vi "Stop AMC Queue.vi"(8 "error in (no error)":errorcluster, 11 "Model_AMC in":refnum<class "Model_AMC.lvclass">) -> (0 "error out":errorcluster, 2 "Exist CMD":string, 3 "Model_AMC out":refnum<class "Model_AMC.lvclass">)   [LabVIEW 2021, in "Model_AMC.lvclass"]
uses:
  Model_AMC.lvclass
  Model_AMC.lvclass/Model_AMC.ctl
  58014273-f04a-4b47-9aff-988d5dec622c.vi
  8ad511de-be0c-4148-9c49-af70c3a993ee.vi
  <vilib>/ActorFramework/Stop Msg/Stop Msg.lvclass
  <vilib>/ActorFramework/Actor/Actor.lvclass
  C:/Program Files (x86)/National Instruments/LabVIEW 2021/user.lib/John_Lib/AbstractActorTemplate/AbstractActorTemplate/UIActorTop.lvclass
  C:/Program Files (x86)/National Instruments/LabVIEW 2021/vi.lib/ActorFramework/Actor/Actor.lvclass
  C:/Program Files (x86)/National Instruments/LabVIEW 2021/project/Create Actor from Template/_Model_AMC/Model_AMC.lvclass
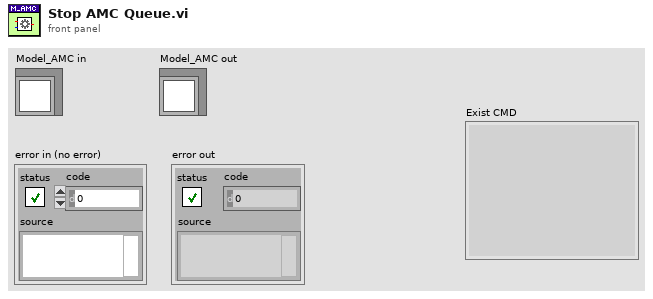
[diagram p1: front panel]
types:
  T1 = typedef "Model_AMC.lvclass/DVR.ctl" = cluster{"JKI_Network_Streams":refnum<class "NetworkConnection.lvclass">, "AMC Q":T2, "Connnected":bool}
  T2 = typedef "Model_AMC.lvclass/AMC Q.ctl" = cluster{"Main":T3, "OPCUA":T3, "NetworkSteam":T3}
  T3 = typedef "AMC_FW.lvlib/Queue.ctl" = cluster{"Q":T4, "Name":string}
  T4 = typedef "AMC_FW.lvlib/Message Queue.ctl" = refnum<queue>
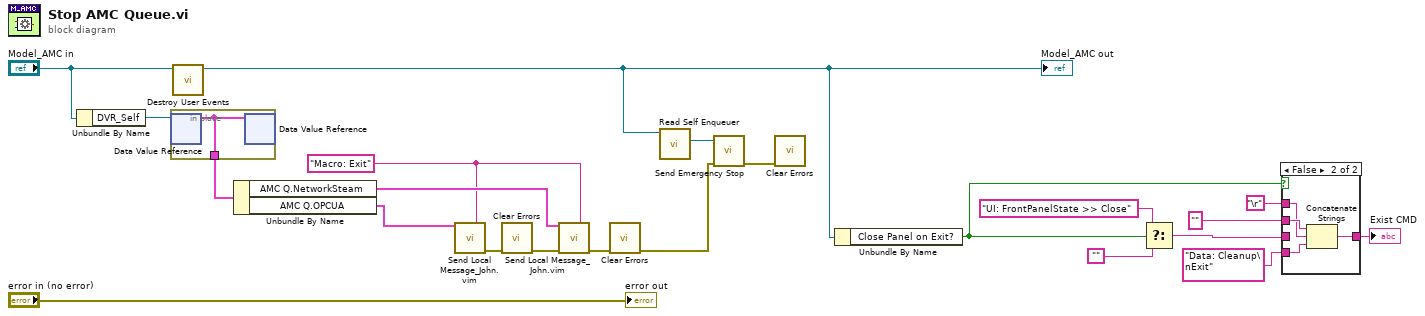
[diagram p0: block diagram]
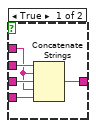
[diagram p2: hidden frame]
diagram:
  w14 = "Macro: Exit" ("Elements in Front")
  n1 = Unbundle By Name("Model_AMC in") -> ("DVR_Self"=w19:refnum<data-value>)
  n2 = in-place {
    in-place-border: [w23] -> w20
    n3 = in-place-dvr #1(w19) -> (w23:T1)  [unwired: 1 out]
    n4 = in-place-dvr #1(w23) -> ()  [unwired: 2 out]
  }
  n5 = call "Destroy User Events.vi"("UI Template in"="Model_AMC in") -> ("UI Template out"=w2:refnum<class "Model_AMC.lvclass">)  [unwired: 10 in]
  "Model_AMC out" <- w2
  n6 = Unbundle By Name(w20) -> ("AMC Q.NetworkSteam"=w21:T3, "AMC Q.OPCUA"=w15:T3)
  n7 = call "Send Local Message_John.vim"("Queue In"=w15, "Elements in Front"=w14) -> ("error out"=w16:errorcluster)  [unwired: 11 in, 2 out]
  n8 = call <vilib>:"Clear Errors.vi"("error in (no error)"=w16) -> ("error out"=w17:errorcluster)  [unwired: 5 in, 1 out]
  n9 = call "Send Local Message_John.vim"("Queue In"=w21, "Elements in Front"=w14, "error in"=w17) -> ("error out"=w18:errorcluster)  [unwired: 10 in, 2 out]
  n10 = call <vilib>:"Clear Errors.vi"("error in (no error)"=w18) -> ("error out"=w4:errorcluster)  [unwired: 5 in, 1 out]
  n11 = call <vilib>:"Read Self Enqueuer.vi"("Actor"=w2) -> ("Self Enqueuer"=w5:refnum<class "Message Enqueuer.lvclass">)  [unwired: 10 in]
  n12 = call <vilib>:"Send Emergency Stop.vi"("error in (no error)"=w4, "Message Enqueuer"=w5) -> ("error out"=w6:errorcluster)  [unwired: 9 in]
  n13 = call <vilib>:"Clear Errors.vi"("error in (no error)"=w6) -> ()  [unwired: 5 in, 2 out]
  n14 = Unbundle By Name(w2) -> ("Close Panel on Exit?"=w7:bool)
  n15 = Select(t="UI: FrontPanelState >> Close", s=w7, f="") -> (s? t:f=w8:string)
  n16 = case shown="False" w7 {
    tunnel: w8 -> [w27 _]
    tunnel: "" -> [w28 w32]
    tunnel: "\r" -> [w26 w31]
    tunnel: "Data: Cleanup\nExit" -> [w25 w30]
    tunnel: [w24 w29] -> w1
    frame True {
      n17 = Concatenate Strings(w28, w26, w27, w26, w25) -> (w24:string)
    }
    frame False {
      n18 = Concatenate Strings(w32, w31, w30) -> (w29:string)
    }
  }
  "Exist CMD" <- w1
  "error out" <- "error in (no error)"
